vi "subHamamatsu_SetROI.vi"(7 "ROI":T1={"Bin"=2, "ROI"={"x offset"=256, "y offset"=256, "x width"=512, "y width"=512}} {"ROI"."x offset" min=1 max=512 step=1; "ROI"."y offset" min=1 max=512 step=1; "ROI"."x width" min=1 max=512 step=1; "ROI"."y width" min=1 max=512 step=1; "Bin" items=["1x1"=1, "2x2"=2, "4x4"=4]}, 8 "error in (no error)":errorcluster, 11 "Handle in":u32) -> (0 "error out":errorcluster, 2 "Sub Region":T2, 3 "Handle out":u32)   [LabVIEW 2015]
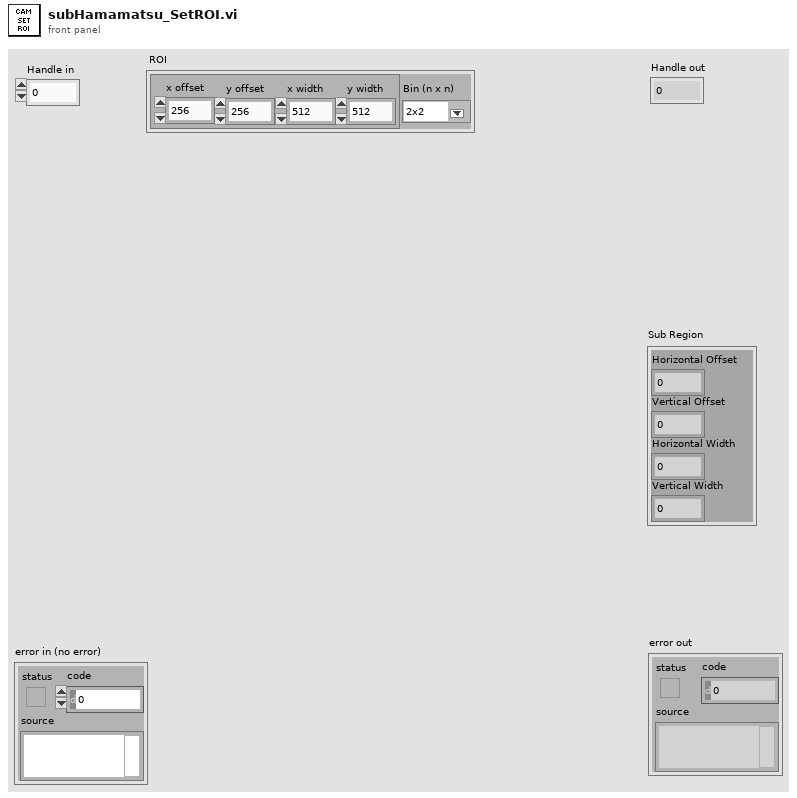
[diagram p1: front panel]
types:
  T1 = cluster{"Bin":u16, "ROI":cluster{"x offset":i32, "y offset":i32, "x width":i32, "y width":i32}}
  T2 = cluster{"Horizontal Offset":i32, "Vertical Offset":i32, "Horizontal Width":i32, "Vertical Width":i32}
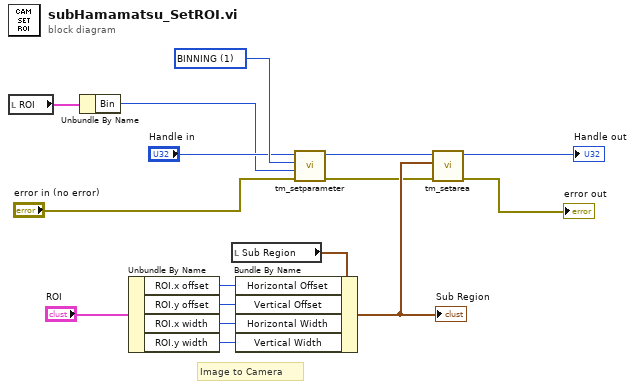
[diagram p0: block diagram]
diagram:
  w9 = 1 items=["BINNING"=1, "BITS PER CHANNEL"=2, "ACTIVE VIEW INDEX"=3, "CCD MODE"=4, "SENSOR MODE"=5, "READOUT MODE"=6, "EXPOSURE TIME"=7, "CONTRAST GAIN"=8, "CONTRAST OFFSET"=9, "LIGHT MODE"=10, "SENSITIVITY"=11, "WHITE BALANCE"=12, "PHOTON IMAGING MODE"=13, "HIGH DYNAMIC RANGE MODE"=14, "TRIGGER SOURCE"=15, "TRIGGER ACTIVE"=16, "TRIGGER MODE"=17, "TRIGGER POLARITY"=18, "TRIGGER GLOBAL EXPOSURE"=19, "FIRST TRIGGER BEHAVIOR"=20, "TRIGGER TIMES"=21, "OUTPUT TRIGGER POLARITY"=22, "OUTPUT TRIGGER DELAY"=23, "OUTPUT TRIGGER PERIOD"=24, "TEMPERATURE"=25, "TEMPERATURE TARGET"=26, "SENSOR COOLER FAN"=27, "MECHANICAL SHUTTER"=28, "BACK FOCUS POSITION"=29, "FRAMEBUNDLE MODE"=30, "FRAMEBUNDLE NUMBER"=31, "LINEBUNDLE HEIGHT"=32, "TRIGGER CONNECTOR"=33, "IMAGE PIXEL TYPE"=34] ("Parameter")
  # "Image to Camera"
  n1 = local read "ROI"() -> (w2:T1)
  n2 = Unbundle By Name(w2) -> ("Bin"=w1:u16)
  n3 = Unbundle By Name("ROI") -> ("ROI.x offset"=w15:i32, "ROI.y offset"=w14:i32, "ROI.x width"=w13:i32, "ROI.y width"=w12:i32)
  n4 = local read "Sub Region"() -> (w16:T2)
  n5 = Bundle By Name(cluster=w16, "Horizontal Offset"=w15, "Vertical Offset"=w14, "Horizontal Width"=w13, "Vertical Width"=w12) -> (w11:T2)
  "Sub Region" <- w11
  n6 = call "tm_setparameter.vi"("error in (no error)"="error in (no error)", "Value in"=w1, "Parameter"=w9, "Handle in"="Handle in") -> ("error out"=w6:errorcluster, "Handle out"=w8:u32)  [unwired: 6 in]
  n7 = call "tm_setarea.vi"("error in (no error)"=w6, "Sub Region"=w11, "Handle in"=w8) -> ("error out"=→"error out":errorcluster, "Handle out"=→"Handle out":u32)  [unwired: 7 in]
